vi "VisionDashRead_General.vi"() -> (0 "PosYFt":dbl, 1 "PosXFt":dbl, 2 "InitOrientDeg":dbl, 3 "InitYFt":dbl, 4 "PosOrientDeg":dbl, 5 "InitXFt":dbl, 6 "OdomErr":bool, 7 "MaxAmbiguity":dbl)   [LabVIEW 2023]
doc: "Vision Network\n\nInput\n --Error in \n\nOutput\n --Error out"
uses:
  <vilib>/Rock Robotics/Network Tables/NT Read Number.vi
  <vilib>/Rock Robotics/Network Tables/NT Read Boolean.vi
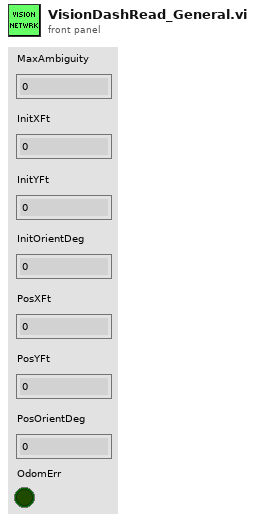
[diagram p1: front panel]
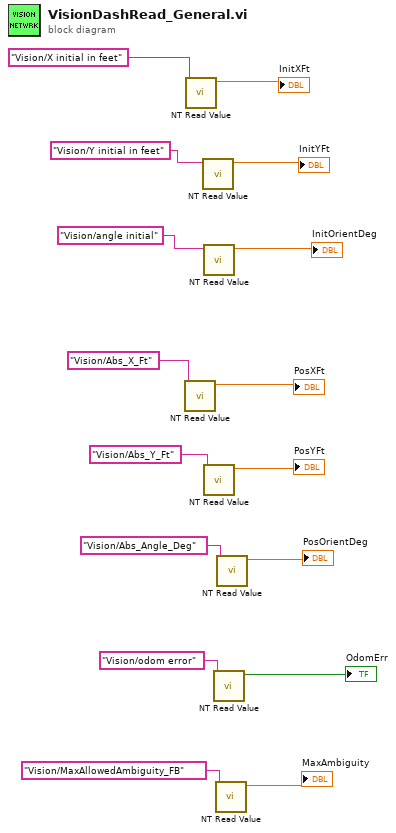
[diagram p0: block diagram]
diagram:
  n1 = call-poly <vilib>:"NT Read Value.vi"("name"="Vision/Abs_X_Ft") -> ("value"=→"PosXFt":dbl)  [unwired: 8 in, 2 out]
  n2 = call-poly <vilib>:"NT Read Value.vi"("name"="Vision/X initial in feet") -> ("value"=→"InitXFt":dbl)  [unwired: 8 in, 2 out]
  n3 = call-poly <vilib>:"NT Read Value.vi"("name"="Vision/Y initial in feet") -> ("value"=→"InitYFt":dbl)  [unwired: 8 in, 2 out]
  n4 = call-poly <vilib>:"NT Read Value.vi"("name"="Vision/angle initial") -> ("value"=→"InitOrientDeg":dbl)  [unwired: 8 in, 2 out]
  n5 = call-poly <vilib>:"NT Read Value.vi"("name"="Vision/Abs_Y_Ft") -> ("value"=→"PosYFt":dbl)  [unwired: 8 in, 2 out]
  n6 = call-poly <vilib>:"NT Read Value.vi"("name"="Vision/odom error") -> ("value"=→"OdomErr":bool)  [unwired: 8 in, 2 out]
  n7 = call-poly <vilib>:"NT Read Value.vi"("name"="Vision/MaxAllowedAmbiguity_FB") -> ("value"=→"MaxAmbiguity":dbl)  [unwired: 8 in, 2 out]
  n8 = call-poly <vilib>:"NT Read Value.vi"("name"="Vision/Abs_Angle_Deg") -> ("value"=→"PosOrientDeg":dbl)  [unwired: 8 in, 2 out]
